vi "test_is_daemon.vi"() -> ()   [LabVIEW 2022 SP3]
uses:
  <instrlib>/yaq/yaq_labview_error_handler.vi
  <vilib>/Utility/error.llb/Simple Error Handler.vi
panel:
  out "path":path
  out "id":string
  out "state":string
  out "config":string
  out "busy?":bool
  in  "Python path":path=path "C:/ProgramData/Anaconda3/envs/lv4/pythonw.exe"
  in  "Python version":string="3.8.0"
  in  "Python Module Path":path=path "C:/Users/kamey/work/labview/yaqc-labview/python/yaqc_labview.py"
  in  "Port":i32=39004
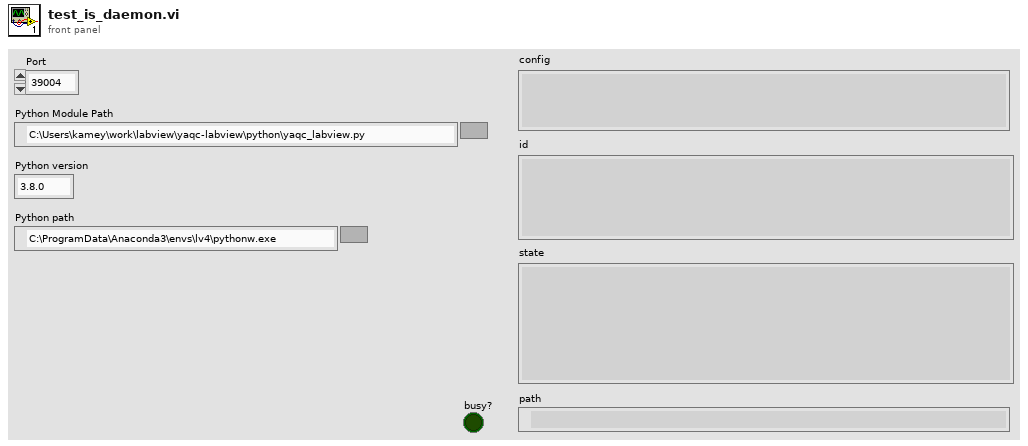
[diagram p1: front panel]
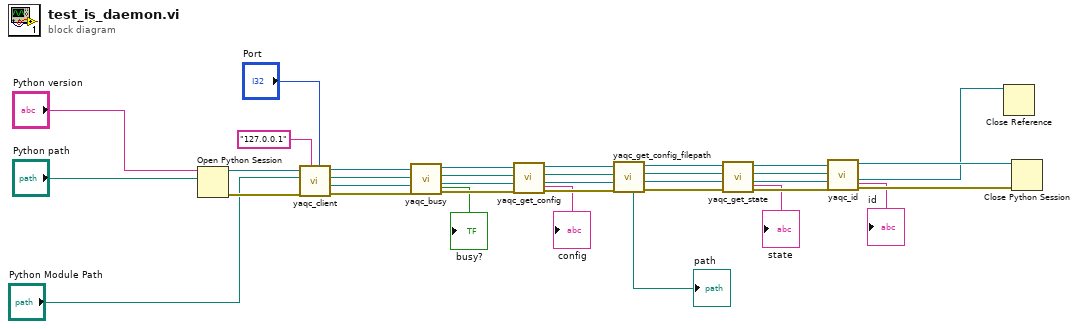
[diagram p0: block diagram]
diagram:
  n1 = Open Python Session(python version="Python version", python path="Python path") -> (session out=w34:refnum<k35>, error out=w35:errorcluster)  [unwired: 1 in]
  n2 = call "yaqc_client.vi"("Port"="Port", "host ('127.0.0.1')"="127.0.0.1", "error in (no error)"=w35, "Python Module Path"="Python Module Path", "Python Session In"=w34) -> ("error out"=w23:errorcluster, "Yaqc Client"=w6:refnum<k38>, "Python Module Path Out"=w15:path, "Python Session Out"=w28:refnum<k35>)  [unwired: 3 in]
  n3 = call <instrlib>:"yaqc_busy.vi"("error in (no error)"=w23, "Yaqc Client In"=w6, "Python Module Path In"=w15, "Python Session In"=w28) -> ("error out"=w22:errorcluster, "Yaqc Client Out"=w7:refnum<k38>, "Python Module Path Out"=w14:path, "Python Session Out"=w27:refnum<k35>, "busy?"=→"busy?":bool)  [unwired: 3 in]
  n4 = call <instrlib>:"yaqc_get_config.vi"("error in (no error)"=w22, "Yaqc Client In"=w7, "Python Module Path In"=w14, "Python Session In"=w27) -> ("error out"=w21:errorcluster, "Yaqc Client Out"=w8:refnum<k38>, "Python Module Path Out"=w13:path, "Python Session Out"=w26:refnum<k35>, "config"=→"config":string)  [unwired: 3 in]
  n5 = call <instrlib>:"yaqc_get_config_filepath.vi"("error in (no error)"=w21, "Yaqc Client In"=w8, "Python Module Path In"=w13, "Python Session In"=w26) -> ("error out"=w20:errorcluster, "Yaqc Client Out"=w9:refnum<k38>, "Python Module Path Out"=w12:path, "Python Session Out"=w25:refnum<k35>, "filepath"=→"path":path)  [unwired: 3 in]
  n6 = call <instrlib>:"yaqc_get_state.vi"("error in (no error)"=w20, "Yaqc Client In"=w9, "Python Module Path In"=w12, "Python Session In"=w25) -> ("error out"=w19:errorcluster, "Yaqc Client Out"=w10:refnum<k38>, "Python Module Path Out"=w11:path, "Python Session Out"=w24:refnum<k35>, "state"=→"state":string)  [unwired: 3 in]
  n7 = call <instrlib>:"yaqc_id.vi"("error in (no error)"=w19, "Yaqc Client In"=w10, "Python Module Path In"=w11, "Python Session In"=w24) -> ("error out"=w17:errorcluster, "Yaqc Client Out"=w16:refnum<k38>, "Python Session Out"=w18:refnum<k35>, "id"=→"id":string)  [unwired: 3 in, 1 out]
  n8 = Close Reference(reference=w16) -> ()  [unwired: 1 in, 1 out]
  n9 = Close Python Session(session in=w18, error in=w17) -> ()  [unwired: 1 out]
